vi "Create Metadata and Aliases.vi"(8 "error in":errorcluster) -> (0 "error out":errorcluster, 4 "log":string)   [LabVIEW 2024]
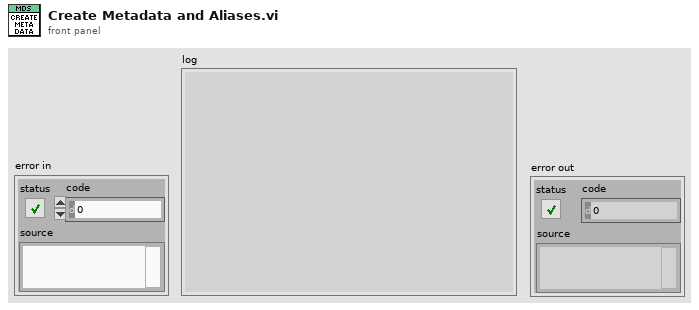
[diagram p1: front panel]
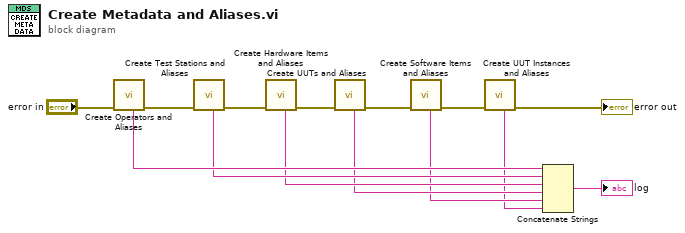
[diagram p0: block diagram]
diagram:
  n1 = call "Create Operators and Aliases.vi"("error in"="error in") -> ("error out"=w14:errorcluster, "log"=w7:string)  [unwired: 9 in]
  n2 = call "Create Test Stations and Aliases.vi"("error in"=w14) -> ("error out"=w13:errorcluster, "log"=w6:string)  [unwired: 9 in]
  n3 = call "Create Hardware Items and Aliases.vi"("error in"=w13) -> ("error out"=w12:errorcluster, "log"=w5:string)  [unwired: 9 in]
  n4 = call "Create UUTs and Aliases.vi"("error in"=w12) -> ("error out"=w11:errorcluster, "log"=w4:string)  [unwired: 9 in]
  n5 = call "Create Software Items and Aliases.vi"("error in"=w11) -> ("error out"=w9:errorcluster, "log"=w3:string)  [unwired: 9 in]
  n6 = call "Create UUT Instances and Aliases.vi"("error in"=w9) -> ("error out"=→"error out":errorcluster, "log"=w2:string)  [unwired: 9 in]
  n7 = Concatenate Strings(w7, w6, w5, w4, w3, w2) -> (→"log":string)
